vi "Topo & GridSpectr_DriftCorrection_v2.vi"(6 "Internal use":string, 7 "Grid param":T2 {"height (m)" format="%#_6p"; "width (m)" format="%#_6p"; "center Y (m)" format="%#_6p"; "center X (m)" format="%#_6p"}, 8 "Error in (no error)":errorcluster, 9 "Points Y/Index Y":i32, 10 "Points X/Index X":i32, 11 "Method":enum16{"init", "run", "end"}(ring)=enum."end") -> (0 "Error out":errorcluster)   [LabVIEW 2014]
doc: "Example of a measurement VI to be used in the \"Experiments on a Grid\" tool as external VI.\n\nThis example measure the topography and spectroscopy data. The spectroscopy measurements are taken on a subgrid. The data are saved to a sxm and a binary file.\n\n- Nanonis Programming Interface -"
uses:
  <userlib>/Nanonis Prog Interface V5/Nanonis Prog Interface.lvlib
panel:
  in  "Drift Correction 2":T1
  out "Numeric":i32
  out "X drift":i32
  out "Y drift":i32
  out "Queue Steps":i32
  in  "StepsBack":i32
  in  "Channel index (0-23)":u8=14
  in  "File name":string
  in  "STS Current":dbl format="%#_6p"
  in  "Imaging Current":dbl format="%#_6p"
  in  "zdrift \nDuration (s)":dbl
  in  "Correct z drift":bool
  out "Status":string="init"
  in  "Drift correction Pixels":i32=128 caption="Pixels for drift correction"
  out "Y Offset":dbl
  out "X Offset":dbl
  out "Points taken":dbl=1.0
  in  "Drift Correction":i32=128
  in  "Y subgrid spacing":u16=1
  in  "X subgrid spacing":u16=1
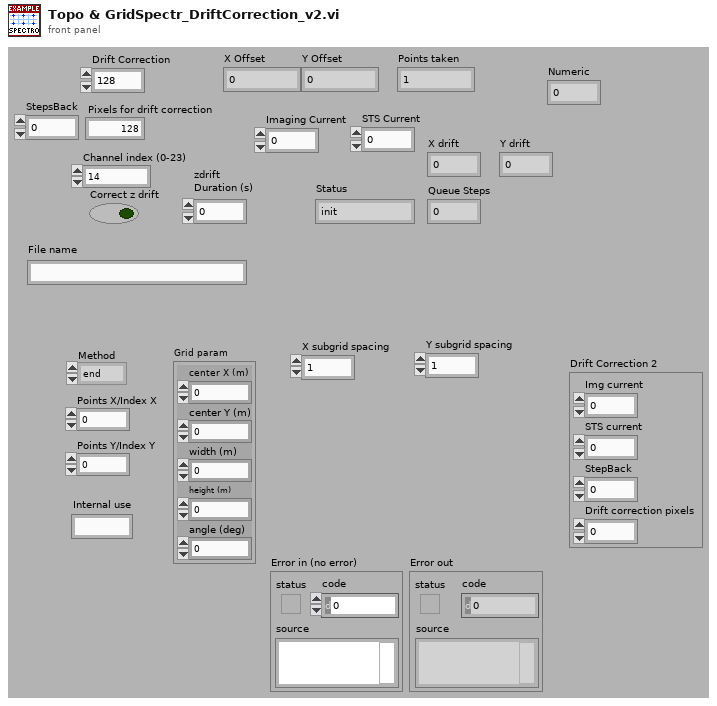
[diagram p1: front panel]
types:
  T1 = cluster{"Img current":dbl, "STS current":dbl, "StepBack":dbl, "Drift correction pixels":dbl}
  T2 = cluster{"center X (m)":sgl, "center Y (m)":sgl, "width (m)":sgl, "height (m)":sgl, "angle (deg)":sgl}
  T3 = enum16{"open", "replace", "create", "open or create", "replace or create", "replace or create with confirmation"}
  T4 = cluster{"center X":sgl, "center Y":sgl, "angle":sgl, "width":sgl, "height":sgl, "# pixels":i32, "# lines":i32}
  T5 = cluster{"Name":string, "Calibration":sgl, "Offset":sgl, "Channel index":i32}[]
  T6 = cluster{"up/down":bool, "time/line":sgl, "start time":timestamp, "end time":timestamp}
  T7 = cluster{"Z averaging time (s)":sgl, "Z offset (m)":sgl, "Initial settling time (s)":sgl}
  T8 = cluster{"Max. slew rate (V/s)":sgl, "Settling time (s)":sgl, "Integration time (s)":sgl}
  T9 = cluster{"End settling time (s)":sgl, "Z control time (s)":sgl}
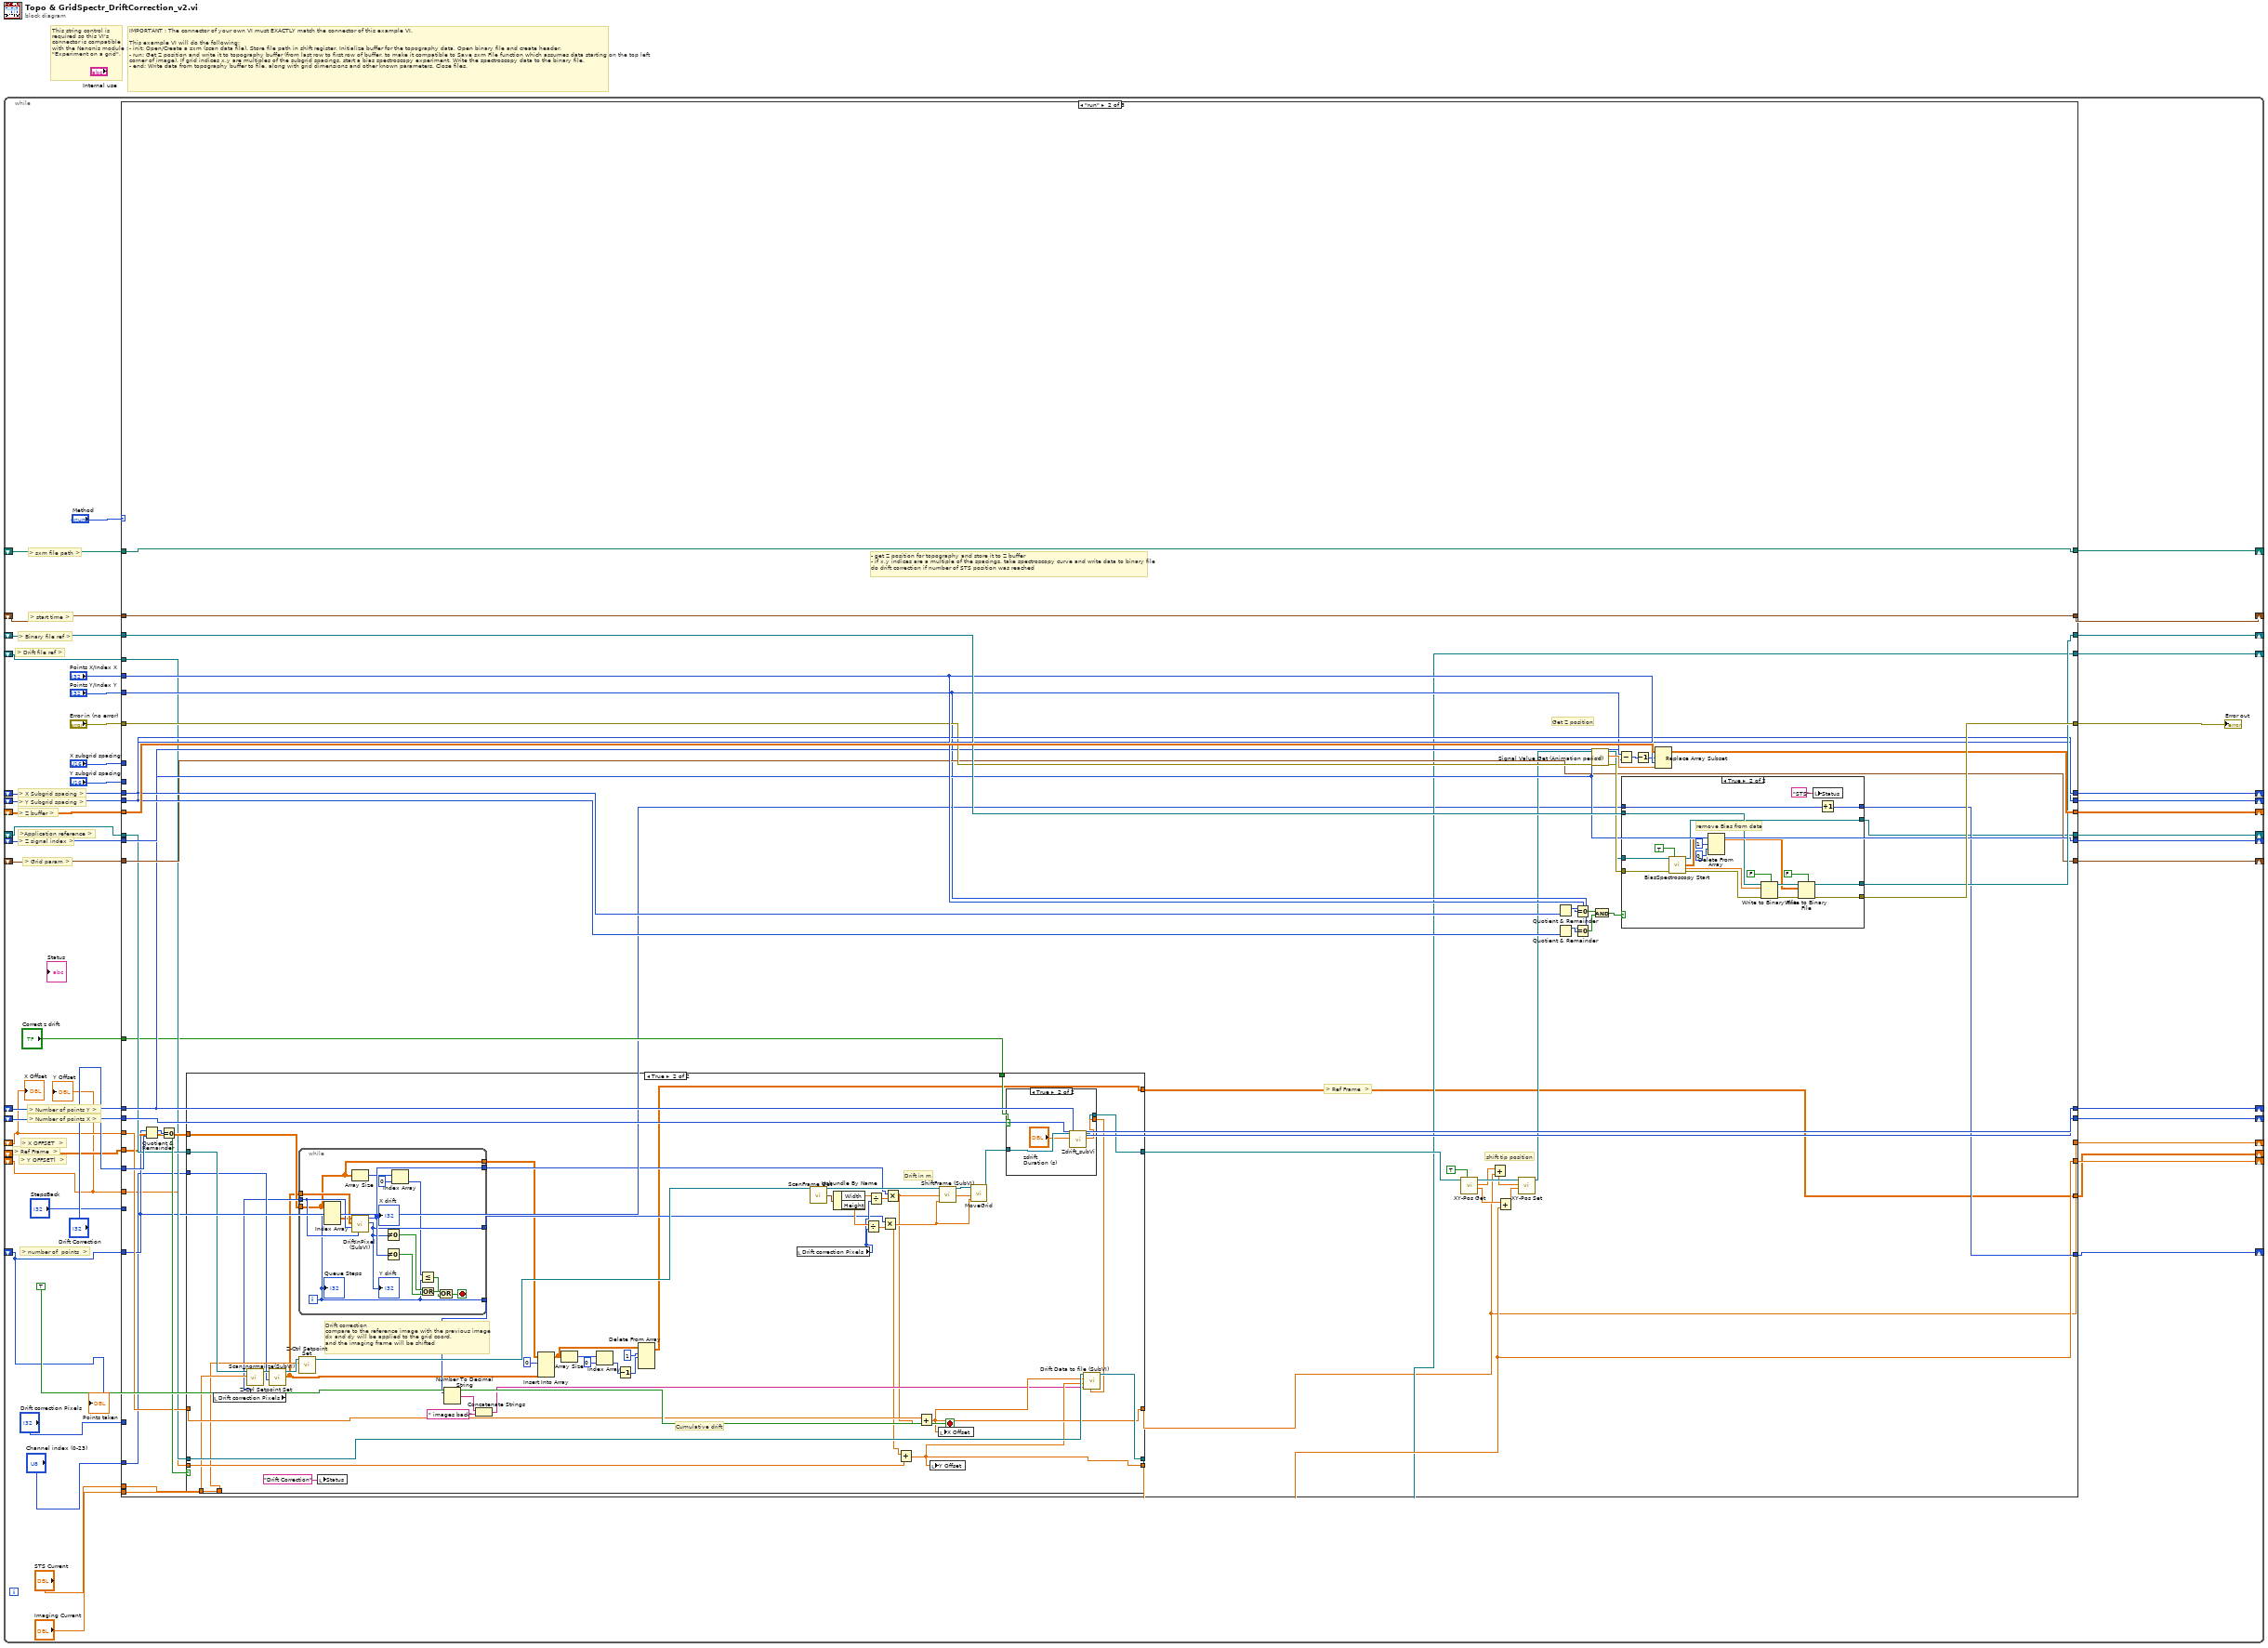
[diagram p0: block diagram]
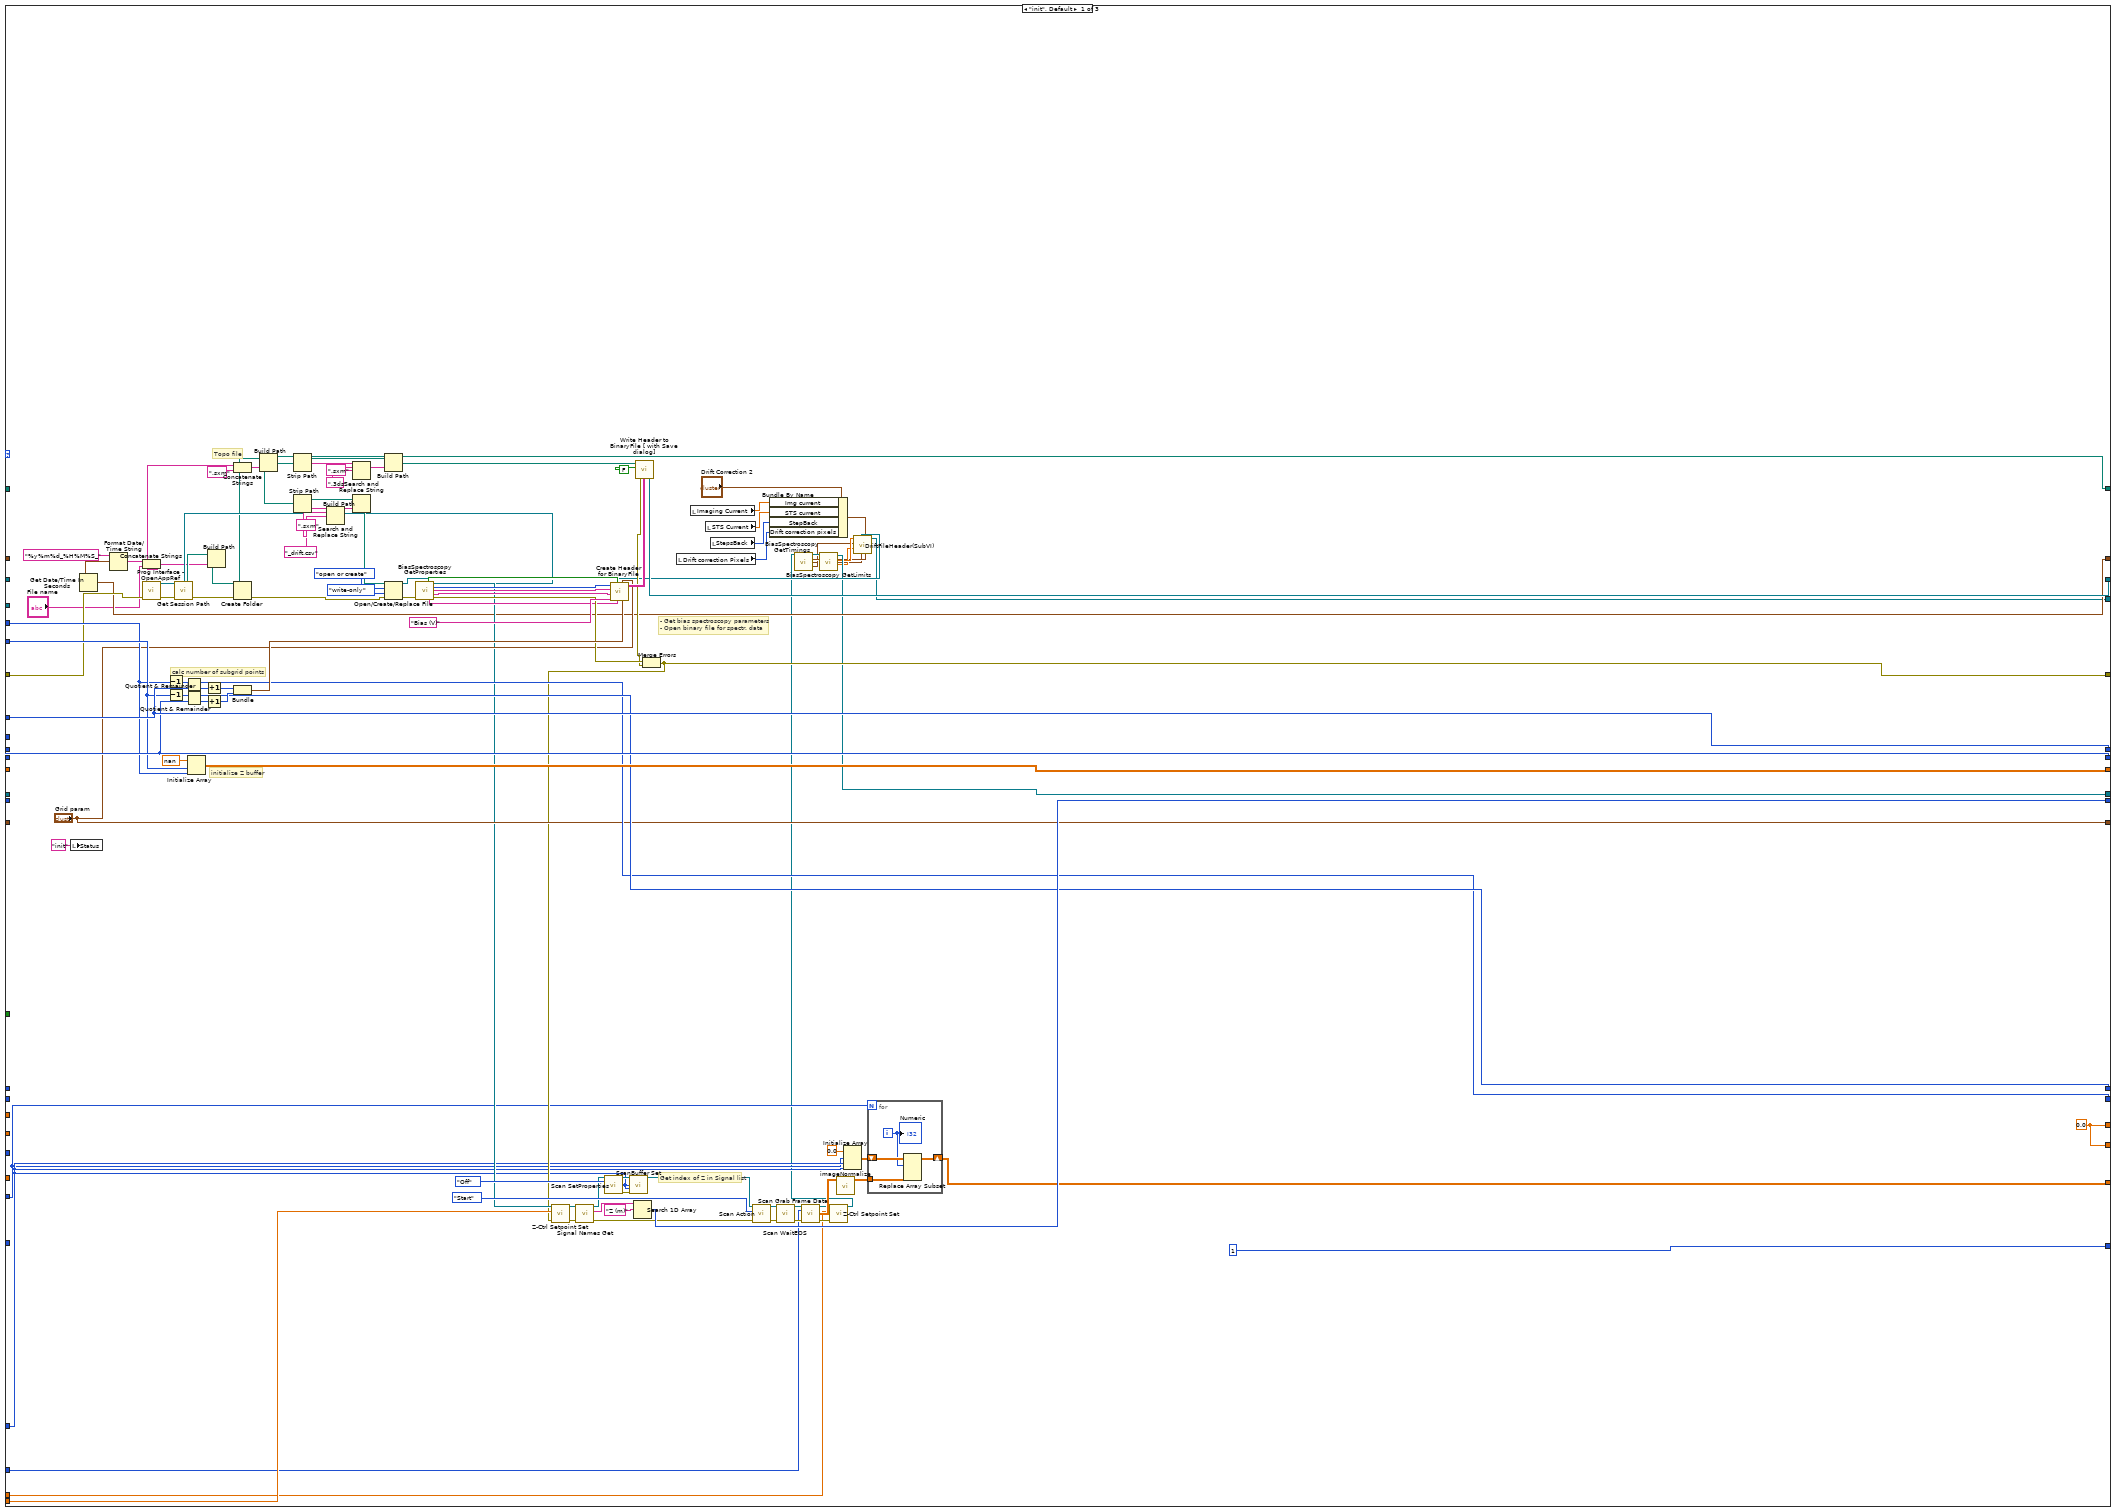
[diagram p2: hidden frame]
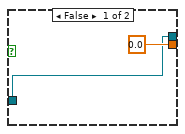
[diagram p4: hidden frame]
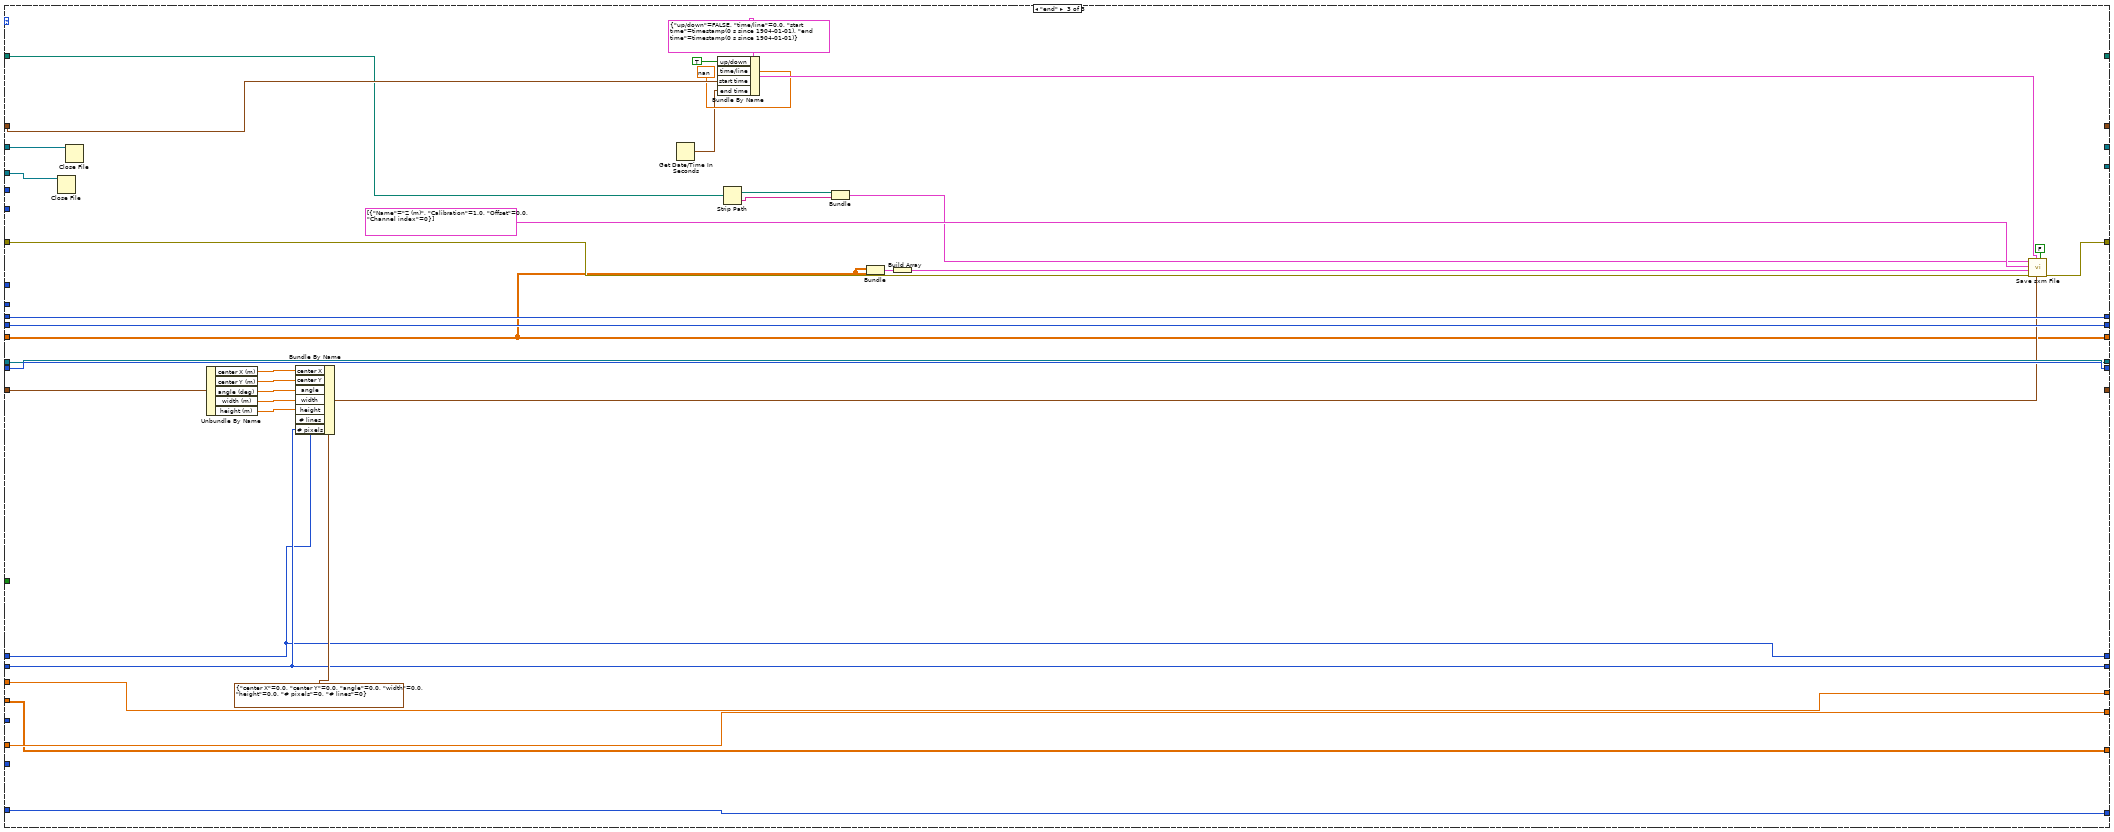
[diagram p6: hidden frame]
diagram:
  # "This string control is required so this VI's connector is compatible with the Nanonis module : \"Experiment on a grid\"."
  # "IMPORTANT : The connector of your own VI must EXACTLY match the connector of this example VI.\n\nThis example VI will do the following:\n- init: Open/Create a sxm (scan data file). Store file path in shift register. Initialize buffer for the topography data. Open binary file and create header.\n- run: Get Z position and write it to topography buffer (from last row to first row of buffer, to make it compatible to Save sxm File function which assumes data starting on the top left corner of image). If grid indices x,y are multiples of the subgrid spacings, start a bias spectroscopy experiment. Write the spectroscopy data to the binary file.\n- end: Write data from topography buffer to file, along with grid dimensions and other known parameters. Close files."
  n1 = while {
    shift-right: [w22] -> _
    shift-left: _ -> [w45]
    shift-right: [w40] -> _
    shift-left: _ -> [w39]
    shift-right: [w37] -> _
    shift-left: _ -> [w38]
    shift-right: [w36] -> _
    shift-left: _ -> [w35]
    shift-right: [w29] -> _
    shift-left: _ -> [w31]
    shift-right: [w30] -> _
    shift-left: _ -> [w32]
    shift-right: [w28] -> _
    shift-left: _ -> [w27]
    shift-right: [w26] -> _
    shift-left: _ -> [w25]
    shift-right: [w24] -> _
    shift-left: _ -> [w23]
    shift-right: [w21] -> _
    shift-left: _ -> [w20]
    shift-right: [w19] -> _
    shift-left: _ -> [w18]
    shift-right: [w17] -> _
    shift-left: _ -> [w10]
    shift-right: [w16] -> _
    shift-left: _ -> [w9]
    shift-right: [w15] -> _
    shift-left: _ -> [w12]
    shift-right: [w14] -> _
    shift-left: _ -> [w11]
    shift-right: [w7] -> _
    shift-left: _ -> [w6]
    stop <- TRUE stop-if-true
    # "> Drift file ref >"
    # "> number of  points  >"
    # "> Ref Frame  >"
    # "> Y OFFSETl  >"
    # "> X OFFSET  >"
    # "> Number of points X >"
    # "> Number of points Y >"
    # "> Grid param >"
    # "> start time >"
    # ">Application reference >"
    # "> Y Subgrid spacing >"
    # "> X Subgrid spacing >"
    # "> Z signal index >"
    # "> Binary file ref >"
    # "> Z buffer >"
    # "> sxm file path >"
    n2 = case shown="\"run\"" "Method" {
      tunnel: [w77 w210 _] -> w22
      tunnel: w45 -> [_ w210 w333]
      tunnel: "Error in (no error)" -> [w84 w196 w326]
      tunnel: [w93 w209 w325] -> w43
      tunnel: "Points X/Index X" -> [w128 w204 _]
      tunnel: "Points Y/Index Y" -> [w129 w188 _]
      tunnel: [w153 w207 w314] -> w40
      tunnel: w39 -> [_ w208 w314]
      tunnel: w38 -> [_ w206 w342]
      tunnel: [w144 w205 _] -> w37
      tunnel: [w142 w194 w343] -> w36
      tunnel: w35 -> [_ w194 w343]
      tunnel: "X subgrid spacing" -> [w141 _ _]
      tunnel: "Y subgrid spacing" -> [w140 _ _]
      tunnel: w32 -> [_ w198 w341]
      tunnel: w31 -> [_ w197 w340]
      tunnel: [w141 w198 w341] -> w30
      tunnel: [w140 w197 w340] -> w29
      tunnel: [w53 w180 w339] -> w28
      tunnel: w27 -> [_ w179 w339]
      tunnel: ["Grid param" w191 _] -> w26
      tunnel: w25 -> [_ w191 w324]
      tunnel: [w74 w192 _] -> w24
      tunnel: w23 -> [_ w192 w334]
      tunnel: [w129 w189 w315] -> w21
      tunnel: w20 -> [_ w189 w315]
      tunnel: [w128 w190 w316] -> w19
      tunnel: w18 -> [_ w190 w316]
      tunnel: [w119 w163 w313] -> w17
      tunnel: [w119 w169 w311] -> w16
      tunnel: [w67 w160 w307] -> w15
      tunnel: [1 w185 w312] -> w14
      tunnel: w11 -> [_ w164 w312]
      tunnel: "Drift Correction" -> [_ w183 _]
      tunnel: w12 -> [_ w168 w307]
      tunnel: w10 -> [_ w181 w313]
      tunnel: w9 -> [_ w158 w311]
      tunnel: "Drift correction Pixels" -> [w66 _ _]
      tunnel: [w62 w166 _] -> w7
      tunnel: w6 -> [_ w167 w308]
      tunnel: "Correct z drift" -> [_ w165 _]
      tunnel: "Imaging Current" -> [w94 w162 _]
      tunnel: "STS Current" -> [w89 w161 _]
      tunnel: "Channel index (0-23)" -> [w70 w159 _]
      tunnel: "StepsBack" -> [w65 _ _]
      frame "init", Default {
        w119 = 0.0
        # "Topo file"
        # "- Get bias spectroscopy parameters\n- Open binary file for spectr. data"
        # "initialize Z buffer"
        # "calc number of subgrid points"
        # "Get index of Z in Signal list"
        n3 = local write "Status"("init" ("Status")) -> ()
        n4 = Get Date/Time In Seconds() -> (seconds since 1Jan1904=w74:timestamp)
        n5 = Format Date/Time String(time format string (%c)="%y%m%d_%H%M%S_", seconds (now)=w74) -> (date/time string=w73:string)  [unwired: 1 in]
        n6 = Concatenate Strings(w73, "File name") -> (w75:string)
        n7 = call <userlib>:"Prog Interface - OpenAppRef.vi"("Error in (no error)"=w84) -> ("Error out"=w86:errorcluster, "Application reference"=w88:refnum<vi>)  [unwired: 5 in]
        n8 = Decrement(x=w128) -> (x-1=w139:i32)
        n9 = Decrement(x=w129) -> (x-1=w138:i32)
        n10 = call <userlib>:"Get Session Path.vi"("error in (no error)"=w86, "Application ref in"=w88) -> ("error out"=w82:errorcluster, "Session path"=w85:path, "Application ref out"=w87:refnum<vi>)  [unwired: 7 in]
        n11 = Quotient & Remainder(x=w139, y=w141) -> (floor(x/y)=w137:i32)  [unwired: 1 out]
        n12 = Quotient & Remainder(x=w138, y=w140) -> (floor(x/y)=w136:i32)  [unwired: 1 out]
        n13 = Initialize Array(sgl nan ("element"), w129, w128) -> (w153:sgl[][])
        n14 = Increment(x=w137) -> (x+1=w135:i32)
        n15 = Increment(x=w136) -> (x+1=w134:i32)
        n16 = Build Path(base path=w85, name or relative path=w75) -> (appended path=w81:path)
        n17 = Create Folder(path (use dialog)=w81, error in=w82) -> (created path=w79:path, error out=w76:errorcluster)  [unwired: 1 in, 1 out]
        n18 = Concatenate Strings(w75, ".sxm" ("pattern")) -> (w78:string)
        n19 = Bundle(w135, w134) -> (w148:cluster{i32, i32})  [unwired: 1 in]
        n20 = Build Path(base path=w79, name or relative path=w78) -> (appended path=w77:path)
        n21 = Strip Path(path=w77) -> (stripped path=w103:path, name=w102:string)
        n22 = Strip Path(path=w77) -> (stripped path=w111:path, name=w108:string)
        n23 = Search and Replace String(input string=w108, search string=".sxm", replace string="_drift.csv" ("replace string (\"\")")) -> (result string=w109:string)  [unwired: 5 in, 3 out]
        n24 = Search and Replace String(input string=w102, search string=".sxm", replace string=".3ds" ("replace string (\"\")")) -> (result string=w104:string)  [unwired: 5 in, 3 out]
        n25 = Build Path(base path=w111, name or relative path=w109) -> (appended path=w110:path)
        n26 = Build Path(base path=w103, name or relative path=w104) -> (appended path=w99:path)
        n27 = Open/Create/Replace File(file path (use dialog)=w110, error in=w76, operation (0:open)=T3."open or create", access (0:read/write)=enum16{"read/write", "read-only", "write-only"}."write-only") -> (refnum out=w63:refnum<file>, error out=w83:errorcluster)  [unwired: 2 in, 1 out]
        n28 = call <userlib>:"BiasSpectroscopy GetProperties.vi"("Application ref in"=w87, "Error in (no error)"=w83) -> ("Backward sweep"=w149:bool, "Application ref out"=w96:refnum<vi>, "Number of points"=w131:i32, "Channels"=w130:string[], "Parameters"=w147:string[], "Fixed parameters"=w133:string[], "Error out"=w146:errorcluster)  [unwired: 5 in, 2 out]
        n29 = call <userlib>:"Create Header for BinaryFile.vi"("Grid points"=w148, "Grid param"="Grid param", "Fixed parameters"=w133, "Backward sweep"=w149, "Sweep signal"="Bias (V)" ("Sweep Signal"), "Parameters"=w147, "Channels"=w130, "Points per sweep"=w131) -> ("Header (fixed attributes)"=w151:string[][])  [unwired: 3 in]
        n30 = call <userlib>:"Write Header to BinaryFile [ with Save dialog].vi"("Fixed Attributes"=w151, "Show Dialog? (T)"=FALSE, "Filename"=w99) -> ("Error out"=w145:errorcluster, "File ref"=w144:refnum<file>)  [unwired: 5 in, 2 out]
        n31 = Merge Errors(w146, w145) -> (w93:errorcluster)
        n32 = call <userlib>:"Z-Ctrl Setpoint Set.vi"("error in (no error)"=w93, "Z Controller setpoint"=w94, "Application ref in"=w96) -> ("error out"=w92:errorcluster, "Application ref out"=w95:refnum<vi>)  [unwired: 7 in]
        n33 = call <userlib>:"Signal Names Get.vi"("error in (no error)"=w92, "Application ref in"=w95) -> ("error out"=w120:errorcluster, "Signals Names"=w132:string[], "Application ref out"=w115:refnum<vi>)  [unwired: 5 in]
        n34 = call <userlib>:"Scan SetProperties.vi"("Application ref in"=w115, "Continuous scan"=enum16{"No change", "On", "Off"}."Off") -> ("Application ref out"=w117:refnum<vi>, "Error out"=w116:errorcluster)  [unwired: 12 in]
        n35 = call <userlib>:"ScanBuffer Set.vi"("Application ref in"=w117, "Pixels"=w66, "Lines"=w66, "error in (no error)"=w116) -> ("Application ref out"=w114:refnum<vi>)  [unwired: 10 in, 1 out]
        n36 = Search 1D Array(1D array=w132, element="Z (m)") -> (index of element=w142:i32)  [unwired: 1 in]
        n37 = local read "Drift correction Pixels"() -> (w57:i32)
        n38 = local read "Imaging Current"() -> (w59:dbl)
        n39 = local read "STS Current"() -> (w58:dbl)
        n40 = local read "StepsBack"() -> (w56:i32)
        n41 = call <userlib>:"Scan Action.vi"("error in (no error)"=w120, "Scan action (Start)"=enum16{"Start", "Stop", "Pause", "Resume"}."Start", "Application ref in"=w114) -> ("error out"=w126:errorcluster, "Application ref out"=w125:refnum<vi>)  [unwired: 6 in]
        n42 = Bundle By Name(cluster="Drift Correction 2", "Img current"=w59, "STS current"=w58, "StepBack"=w56, "Drift correction pixels"=w57) -> (w60:T1)
        n43 = call <userlib>:"Scan WaitEOS.vi"("error in (no error)"=w126, "Application ref in"=w125) -> ("error out"=w123:errorcluster, "Application ref out"=w124:refnum<vi>)  [unwired: 5 in, 2 out]
        n44 = call <userlib>:"Scan Grab Frame Data.vi"("Application ref in"=w124, "Channel index (0-23)"=w70, "error in (no error)"=w123) -> ("Application ref out"=w91:refnum<vi>, "Scan frame data"=w97:sgl[][], "error out"=w90:errorcluster)  [unwired: 8 in, 2 out]
        n45 = call <userlib>:"Z-Ctrl Setpoint Set.vi"("error in (no error)"=w90, "Z Controller setpoint"=w89, "Application ref in"=w91) -> ("Application ref out"=w54:refnum<vi>)  [unwired: 7 in, 1 out]
        n46 = call <userlib>:"BiasSpectroscopy GetTimings.vi"("Application ref in"=w54) -> ("Application ref out"=w55:refnum<vi>, "Initialization"=w50:T7, "Sweep Timing"=w48:T8, "End of Sweep"=w49:T9)  [unwired: 10 in, 1 out]
        n47 = call <userlib>:"BiasSpectroscopy GetLimits.vi"("Application ref in"=w55) -> ("End value (V)"=w51:sgl, "Start value (V)"=w52:sgl, "Application ref out"=w53:refnum<vi>)  [unwired: 5 in, 1 out]
        n48 = call "imageNormalize.vi"("Data"=w97) -> ("Array"=w64:dbl[][])  [unwired: 10 in]
        n49 = Initialize Array(0.0 ("element"), w65, w66, w66) -> (w68:dbl[][][])
        n50 = call "DriftFileHeader(SubVI).vi"("Initialization"=w50, "Drift Correction"=w60, "Sweep Timing"=w48, "Byte Stream File in"=w63, "End value (V)"=w51, "End of Sweep"=w49, "Start value (V)"=w52) -> ("Byte Stream File out"=w62:refnum<file>)  [unwired: 4 in]
        n51 = for {
          N: w65 -> [_]
          tunnel: w64 -> [w156]
          shift-right: [w155] -> w67
          shift-left: w68 -> [w157]
          i -> [w154]
          n52 = Replace Array Subset(array=w157, new element=w156, index (dim 0)=w154) -> (w155:dbl[][][])  [unwired: 2 in]
          "Numeric" <- w154
        }
      }
      frame "run" {
        # "> Ref Frame  >"
        # "shift tip position"
        # "Get Z position"
        # "- get Z position for topography and store it to Z buffer\n- if x,y indices are a multiple of the spacings, take spectroscopy curve and write data to binary file\ndo drift correction if number of STS position was reached"
        n53 = Quotient & Remainder(x=w164, y=w183) -> (x-y*floor(x/y)=w184:i32)  [unwired: 1 out]
        n54 = Equal To 0?(x=w184) -> (x = 0?=w182:bool)
        n55 = case shown="True" w182 {
          tunnel: w179 -> [w215 w246]
          tunnel: [w215 w252] -> w178
          tunnel: w168 -> [w212 w234]
          tunnel: [w214 w248] -> w163
          tunnel: [w213 w247] -> w169
          tunnel: w181 -> [w214 w250]
          tunnel: w158 -> [w213 w251]
          tunnel: [w212 w226] -> w160
          tunnel: w167 -> [w211 w255]
          tunnel: [w211 w254] -> w166
          tunnel: w165 -> [_ w249]
          tunnel: w162 -> [_ w245]
          tunnel: w161 -> [_ w243]
          tunnel: w159 -> [_ w238]
          frame False {
          }
          frame True {
            # "Cumulative drift"
            # "Drift in m"
            # "Drift correction \ncompare to the reference image with the previous image \ndx and dy will be applied to the grid coord, \nand the imaging frame will be shifted"
            n56 = local read "Drift correction Pixels"() -> (w237:i32)
            n57 = call <userlib>:"Z-Ctrl Setpoint Set.vi"("Z Controller setpoint"=w245, "Application ref in"=w246) -> ("Application ref out"=w242:refnum<vi>)  [unwired: 8 in, 1 out]
            n58 = call "Scan_normailze(SubVI).vi"("Channel index (0-23)"=w238, "Application in"=w242) -> ("Array"=w228:dbl[][], "Application out"=w244:refnum<vi>)  [unwired: 7 in, 1 out]
            n59 = while {
              tunnel: w237 -> [w274]
              tunnel: w228 -> [w273]
              tunnel: w234 -> [w263]
              tunnel: [w272] -> w236
              tunnel: [w271] -> w235
              tunnel: [w267] -> w233
              tunnel: [w263] -> w229
              i -> [w267]
              stop <- w269 stop-if-true
              n60 = Index Array(array=w263, index (dim 0)=w267) -> (element=w262:dbl[][])  [unwired: 2 in]
              n61 = Array Size(array=w263) -> (size(s)=w266:i32[])
              n62 = call "DriftInPixel (SubVI).vi"(6:w274, 9:w274, "New image"=w273, "Ref image"=w262) -> ("Y drift"=w271:i32, "X drift"=w272:i32)  [unwired: 5 in, 1 out]
              "Y drift" <- w271
              "X drift" <- w272
              n63 = Not Equal To 0?(x=w271) -> (x != 0?=w276:bool)
              n64 = Not Equal To 0?(x=w272) -> (x != 0?=w275:bool)
              n65 = Index Array(array=w266, index=0) -> (element=w264:i32)
              n66 = Less Or Equal?(x=w264, y=w267) -> (x <= y?=w268:bool)
              n67 = Or(x=w276, y=w275) -> (x .or. y?=w270:bool)
              n68 = Or(x=w270, y=w268) -> (x .or. y?=w269:bool)
              "Queue Steps" <- w267
            }
            n69 = call <userlib>:"Z-Ctrl Setpoint Set.vi"("Z Controller setpoint"=w243, "Application ref in"=w244) -> ("Application ref out"=w240:refnum<vi>)  [unwired: 8 in, 1 out]
            n70 = local write "Status"("Drift Correction" ("Status")) -> ()
            n71 = Number To Decimal String(number=w233) -> (decimal integer string=w232:string)  [unwired: 1 in]
            n72 = Concatenate Strings(w232, " images back" ("string")) -> (w231:string)
            n73 = Insert Into Array(array=w229, index (dim 0)=0 ("index (page)"), new element=w228) -> (w225:dbl[][][])  [unwired: 2 in]
            n74 = Array Size(array=w225) -> (size(s)=w224:i32[])
            n75 = Index Array(array=w224, index=0) -> (element=w222:i32)
            n76 = Decrement(x=w222) -> (x-1=w221:i32)
            n77 = Delete From Array(array=w225, length=1, index (dim 0)=w221) -> (array with subset deleted=w226:dbl[][][])  [unwired: 2 in, 1 out]
            n78 = local read "Drift correction Pixels"() -> (w239:i32)
            n79 = call <userlib>:"ScanFrame Get.vi"("Application ref in"=w240) -> ("Application ref out"=w241:refnum<vi>, "Size (m)"=w260:cluster{"Width":sgl, "Height":sgl})  [unwired: 10 in, 3 out]
            n80 = Unbundle By Name(w260) -> ("Width"=w259:sgl, "Height"=w261:sgl)
            n81 = Divide(x=w261, y=w239) -> (x/y=w257:sgl)
            n82 = Divide(x=w259, y=w239) -> (x/y=w258:sgl)
            n83 = Multiply(x=w235, y=w257) -> (x*y=w217:sgl)
            n84 = Multiply(x=w236, y=w258) -> (x*y=w216:sgl)
            n85 = Add(x=w217, y=w251) -> (x+y=w247:dbl)
            n86 = Add(x=w250, y=w216) -> (x+y=w248:dbl)
            n87 = local write "Y Offset"(w247) -> ()
            n88 = local write "X Offset"(w248) -> ()
            n89 = call "ShiftFrame (SubVI).vi"("Y shift"=w217, "X shift"=w216, "Application in"=w241) -> ("Application out"=w219:refnum<vi>)  [unwired: 8 in]
            n90 = call "MoveGrid.vi"("y"=w217, "x"=w216, "Application ref in"=w219) -> ("Application ref out"=w218:refnum<vi>)  [unwired: 7 in, 1 out]
            n91 = case shown="True" w249 {
              tunnel: [0.0 ("z drift") w282] -> w253
              tunnel: w218 -> [w277 w281]
              tunnel: [w277 w280] -> w252
              frame False {
              }
              frame True {
                n92 = call "Zdrift_subVi.vi"("Duration"="zdrift \nDuration (s)", "Application in"=w281) -> ("z drift"=w282:dbl, "Application out"=w280:refnum<vi>)  [unwired: 7 in, 1 out]
              }
            }
            n93 = call "Drift Data to file (SubVI).vi"("z drift"=w253, "Comment"=w231, "y Drift"=w247, "X drift"=w248, "Byte Stream File in"=w255) -> ("Byte Stream File out"=w254:refnum<file>)  [unwired: 6 in]
          }
        }
        n94 = call <userlib>:"XY-Pos Get.vi"("Wait for newest data (F=False)"=TRUE, "Application ref in"=w178) -> ("Y (m)"=w173:sgl, "X (m)"=w174:sgl, "Application ref out"=w175:refnum<vi>)  [unwired: 5 in, 1 out]
        n95 = Add(x=w174, y=w163) -> (x+y=w172:dbl)
        n96 = Add(x=w173, y=w169) -> (x+y=w171:dbl)
        n97 = call <userlib>:"XY-Pos Set.vi"("Y (m)"=w171, "X (m)"=w172, "Application ref in"=w175) -> ("Application ref out"=w176:refnum<vi>)  [unwired: 5 in, 1 out]
        n98 = Quotient & Remainder(x=w204, y=w198) -> (x-y*floor(x/y)=w203:i32)  [unwired: 1 out]
        n99 = Quotient & Remainder(x=w188, y=w197) -> (x-y*floor(x/y)=w202:i32)  [unwired: 1 out]
        n100 = Equal To 0?(x=w203) -> (x = 0?=w201:bool)
        n101 = Equal To 0?(x=w202) -> (x = 0?=w200:bool)
        n102 = call <userlib>:"Signal Value Get (Animation period).vi"("error in (no error)"=w196, "Signal index (0-47)"=w194, "Application ref in"=w176) -> ("error out"=w195:errorcluster, "Signal value"=w193:sgl, "Application ref out"=w177:refnum<vi>)  [unwired: 5 in]
        n103 = And(x=w201, y=w200) -> (x .and. y?=w199:bool)
        n104 = Subtract(x=w189, y=w188) -> (x-y=w187:i32)
        n105 = case shown="True" w199 {
          tunnel: [w285 w290] -> w209
          tunnel: w206 -> [w286 w306]
          tunnel: [w286 w304] -> w205
          tunnel: w195 -> [w285 w303]
          tunnel: w177 -> [w284 w295]
          tunnel: [w284 w294] -> w180
          tunnel: [w283 w288] -> w185
          tunnel: w164 -> [w283 w289]
          frame False {
            # "Point indices aren't multiple of subgrid spacing\n=> no spectroscopy at this point"
          }
          frame True {
            # "remove Bias from data"
            n106 = call <userlib>:"BiasSpectroscopy Start.vi"("Application ref in"=w295, "Get data (F)"=TRUE ("Get Data (F)"), "Error in (no error)"=w303) -> ("Application ref out"=w294:refnum<vi>, "Data"=w302:sgl[][], "Parameters"=w301:sgl[], "Error out"=w292:errorcluster)  [unwired: 8 in, 1 out]
            n107 = Delete From Array(array=w302, length=1, index (row)=0 ("index")) -> (array with subset deleted=w300:sgl[][])  [unwired: 1 in, 1 out]
            n108 = Write to Binary File(file (use dialog)=w306, data=w301, error in=w292, 5:FALSE ("prepend array or string size? (T)")) -> (refnum out=w305:refnum<file>, error out=w291:errorcluster)  [unwired: 2 in, 1 out]
            n109 = Write to Binary File(file (use dialog)=w305, data=w300, error in=w291, 5:FALSE ("prepend array or string size? (T)")) -> (refnum out=w304:refnum<file>, error out=w290:errorcluster)  [unwired: 2 in, 1 out]
            n110 = local write "Status"("STS" ("Status")) -> ()
            n111 = Increment(x=w289) -> (x+1=w288:i32)
          }
        }
        n112 = Decrement(x=w187) -> (x-1=w186:i32)
        n113 = Replace Array Subset(array=w208, new element=w193, index (row)=w186, index (col)=w204) -> (w207:sgl[][])
      }
      frame "end" {
        n114 = Close File(refnum=w308) -> ()  [unwired: 1 in, 2 out]
        n115 = Close File(refnum=w342) -> ()  [unwired: 1 in, 2 out]
        n116 = Unbundle By Name(w324) -> ("center X (m)"=w322:sgl, "center Y (m)"=w321:sgl, "angle (deg)"=w320:sgl, "width (m)"=w319:sgl, "height (m)"=w318:sgl)
        n117 = Bundle By Name(cluster=T4 {"center X"=0.0, "center Y"=0.0, "angle"=0.0, "width"=0.0, "height"=0.0, "# pixels"=0, "# lines"=0} ("Scanfield"), "center X"=w322, "center Y"=w321, "angle"=w320, "width"=w319, "height"=w318, "# lines"=w315, "# pixels"=w316) -> (w317:T4)
        n118 = Get Date/Time In Seconds() -> (seconds since 1Jan1904=w310:timestamp)
        n119 = Bundle By Name(cluster=T6 {"up/down"=FALSE, "time/line"=0.0, "start time"=timestamp(0 s since 1904-01-01), "end time"=timestamp(0 s since 1904-01-01)} ("Scan param"), "up/down"=TRUE, "time/line"=sgl nan ("input 7"), "start time"=w334, "end time"=w310) -> (w332:T6)
        n120 = Strip Path(path=w333) -> (stripped path=w329:path, name=w328:string)
        n121 = Bundle("stripped path"=w329, "name"=w328) -> (w327:cluster{"stripped path":path, "name":string})  [unwired: 1 in]
        n122 = Bundle(w314, w314) -> (w338:cluster{sgl[][], sgl[][]})  [unwired: 1 in]
        n123 = Build Array(w338) -> (w337:cluster{sgl[][], sgl[][]}[])
        n124 = call <userlib>:"Save sxm File.vi"("Auto file naming? (T)"=FALSE, "Scanfield"=w317, "Scan param"=w332, "error in (no error)"=w326, "Channels data"=w337, "Channels config"=T5 [{"Name"="Z (m)", "Calibration"=1.0, "Offset"=0.0, "Channel index"=0}], "Filename control"=w327) -> ("error out"=w325:errorcluster)  [unwired: 2 in, 2 out]
      }
    }
    "Error out" <- w43
    "Points taken" <- w11
    "X Offset" <- w10
    "Y Offset" <- w9
  }
